vi "PI Update Sequence.vi"(8 "error in (no error)":errorcluster, 11 "params":variant) -> (0 "Axis":i32, 3 "Position ACT":dbl)   [LabVIEW 2020]
uses:
  Single Ch PI Position.ctl
  Low Level/Communication.llb/Global1.vi
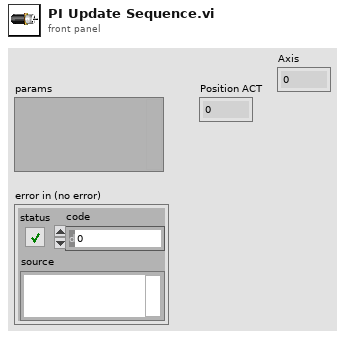
[diagram p1: front panel]
types:
  T1 = typedef "Single Ch PI Position.ctl" = cluster{"Position (SET)":cluster{"XaxesSET":dbl}, "Position (ACT)":cluster{"PosXACT":dbl}}
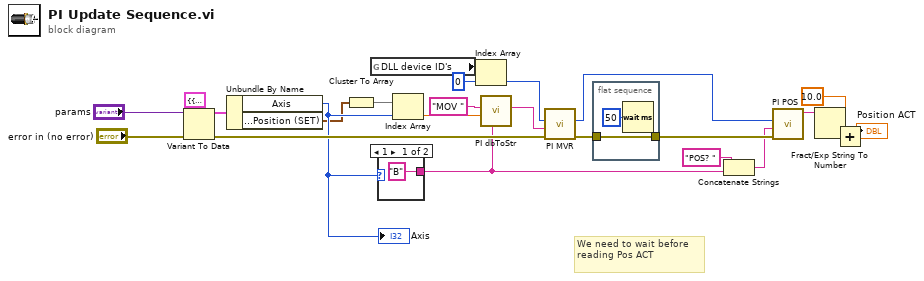
[diagram p0: block diagram]
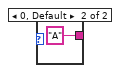
[diagram p2: hidden frame]
diagram:
  # "We need to wait before reading Pos ACT"
  n1 = Variant To Data(error in="error in (no error)", type=cluster{"PIFOC Position":T1, "Axis":i32} {"PIFOC Position"={"Position (SET)"={"XaxesSET"=0.0}, "Position (ACT)"={"PosXACT"=26.9419}}, "Axis"=0} ("input cluster"), Variant="params") -> (data=w22:cluster{"PIFOC Position":T1, "Axis":i32}, error out=w24:errorcluster)
  n2 = Unbundle By Name(w22) -> ("Axis"=w10:i32, "PIFOC Position.Position (SET)"=w6:cluster{"XaxesSET":dbl})
  "Axis" <- w10
  n3 = Cluster To Array(cluster=w6) -> (array=w5:dbl[])
  n4 = global read "Global1.vi" "DLL device ID's"() -> (w19:i32[])
  n5 = case shown="1" w10 {
    tunnel: ["B" "A"] -> w4
    frame 1 {
    }
    frame 0, Default {
    }
  }
  n6 = Index Array(array=w5, index=w10) -> (element=w11:dbl)
  n7 = Index Array(array=w19, index=0) -> (element=w20:i32)
  n8 = call "PI dbToStr.vi"("Axes"=w4, "Start"=w11, "String in"="MOV ") -> ("String out"=w13:string)  [unwired: 8 in]
  n9 = call "PI MVR.vi"("error in (no error)"=w24, "String"=w13, "PI ID in"=w20) -> ("error out"=w15:errorcluster, "PI ID out"=w3:i32)  [unwired: 6 in, 1 out]
  n10 = flat-sequence {
    tunnel: w15 -> [w28]
    tunnel: [w28] -> w16
    frame #0 {
      n11 = Wait (ms)(milliseconds to wait=u32 50 ("Post Wait")) -> ()  [unwired: 1 out]
    }
  }
  n12 = Concatenate Strings("POS? ", w4) -> (w7:string)
  n13 = call "PI POS.vi"("error in (no error)"=w16, "query"=w7, "ID"=w3) -> ("Answer"=w17:string)  [unwired: 6 in, 2 out]
  n14 = Fract/Exp String To Number(string=w17) -> (number=w18:dbl)  [unwired: 3 in, 1 out]
  n15 = Add(x=w18, y=10.0) -> (x+y=→"Position ACT":dbl)
